vi "Project_2_VI.vi"() -> ()   [LabVIEW 2018]
doc: "I. Description:\nThis example demonstrates how to continuously acquire and generate data at the same time, synchronized with one another.\n\nII. Instructions for Running:\n1. Select the physical channel to correspond to where your signal is input on the DAQ device. Also, select the corresponding channel for where your signal is being generated.\n2. Enter the minimum and maximum voltage ranges.\nNote: For better accuracy try to match the input range to the expected voltage level of the measured signal.\n3. Set the sample rate of the acquisition.\nNote: The rate should be at least twice as fast as the maximum frequency component of the signal being acquired. \n6. Select the Rate for the generation\n7. Select what type of signal to generate and the amplitude.\nNote: This example requires two DMA channels to run. If your hardware does not support two DMA channels, you need to set the Data Transfer Mechanism property for the Analog Output Task to use \"Interrupts\". The Data Transfer Mechanism property is located in the DAQmx Channel Property hierarchy at:\n\nDAQmx Channel Property Node>>Analog Output>>General Properties>>Advanced>>Data Transfer and Memory>>Data Transfer Mechanism\n\nRefer to your device documentation to determine how many DMA channels are supported for your hardware.\n\nIII. Block Diagram Steps:\n1. Create an analog input voltage channel. Also, create an analog output voltage channel.\n2. Set the rate for the sample clock. Additionally, define the sample mode to be continuous. Also, set the sample clock rate for the signal generation.\n2a. Call the Get Terminal Name with Device Prefix VI. This will take a Task and a terminal and create a properly formatted device + terminal name to use as the source of the Trigger.\n3. Define the parameters for a Digital Edge Start Trigger. Set the Analog output to trigger off the AI Start Trigger. This is an internal trigger signal.\n4. Use the Basic Function Generator VI to create the signal to be generated.\n5. Call the Start VI to arm the two functions. Make sure the analog output is armed before the analog input. This will ensure both will start at the same time.\n6. Read the waveform data in a loop until the user hits the stop button or an error occurs. The Is Task Done? VI is used to check for errors in the Analog Output Task.\n7. Call the Clear VI to Clear the Task\n8. Use the popup dialog box to display an error if any.\n\nIV. I/O Connections Overview:\nMake sure your signal input/output terminals match the Physical Channel I/O controls."
uses:
  <vilib>/Analysis/4window.llb/windowTd.ctl
  <vilib>/Utility/error.llb/DialogType.ctl
  <vilib>/DAQmx/write.llb/DAQmx Write (Analog Wfm 1Chan NSamp).vi
  <vilib>/DAQmx/read.llb/DAQmx Read (Analog 1D Wfm NChan NSamp).vi
  <vilib>/DAQmx/create/channels.llb/DAQmx Create Channel (AI-Voltage-Basic).vi
  <vilib>/DAQmx/configure/timing.llb/DAQmx Timing (Sample Clock).vi
  <vilib>/DAQmx/create/channels.llb/DAQmx Create Channel (AO-Voltage-Basic).vi
  <vilib>/DAQmx/configure/trigger.llb/DAQmx Start Trigger (Digital Edge).vi
  <vilib>/DAQmx/miscellaneous.llb/DAQmx Fill In Error Info.vi
  <vilib>/Utility/file.llb/Write To Spreadsheet File (DBL).vi
  <vilib>/measure/maspectr.llb/FFT Spectrum (Mag-Phase) for 1 Chan.vi
  <vilib>/Utility/file.llb/Write Delimited Spreadsheet (DBL).vi
  <resource>/objmgr/daqmx.rc
  <vilib>/Analysis/NI_AALBase.lvlib
  <vilib>/measure/NI_MAPro.lvlib
  <vilib>/Analysis/NI_AALPro.lvlib
panel:
  in  "Frequency Response fike path":path=path "E:/Project2/Response.txt"
  in  "averaging parameters":T1={"averaging mode"=enum."No averaging", "weighting mode"=enum."Exponential", "number of averages"=10} {"number of averages" min=1}
  out "Phase Response":cluster{"f0":dbl, "df":dbl, "magnitude":dbl[]}(graph)
  out "Frequency Response":cluster{"f0":dbl, "df":dbl, "magnitude":dbl[]}(graph)
  in  "window":T2 items=["Rectangle"=0, "Hanning"=1, "Hamming"=2, "Blackman-Harris"=3, "Exact Blackman"=4, "Blackman"=5, "Flat Top"=6, "4 Term B-Harris "=7, "7 Term B-Harris"=8, "Low Sidelobe"=9, "Blackman Nuttall"=11, "Triangle"=30, "Bartlett-Hanning"=31, "Bohman"=32, "Parzen"=33, "Welch"=34, "Kaiser"=60, "Dolph-Chebyshev"=61, "Gaussian"=62]
  in  "End frequency (Hz)":dbl=10000.0 format="%.2p"
  in  "Waveform file path":path=path "E:/Project2/data.txt"
  in  "Start frequency":dbl=100.0 format="%0.2p"
  out "Time Domain":waveform(dbl)[](graph)
  in  "Sampling Info":T3={"Sampling Rate"=20000.0, "Number of Samples"=2000} {"Sampling Rate" format="%.2p"}
  in  "Amplitude":dbl=2.0 format="%0.2p"
  in  "Channel":tag="Dev1/ao0" caption="Output Physical Channels"
  in  "Channel":tag="Dev1/ai6,Dev1/ai13" caption="Input Physical Channel"
  # "Channel Parameters"
  # "Signal Generation"
  # "ReIm"
  # "MagPhase"
  # "FRF parameters"
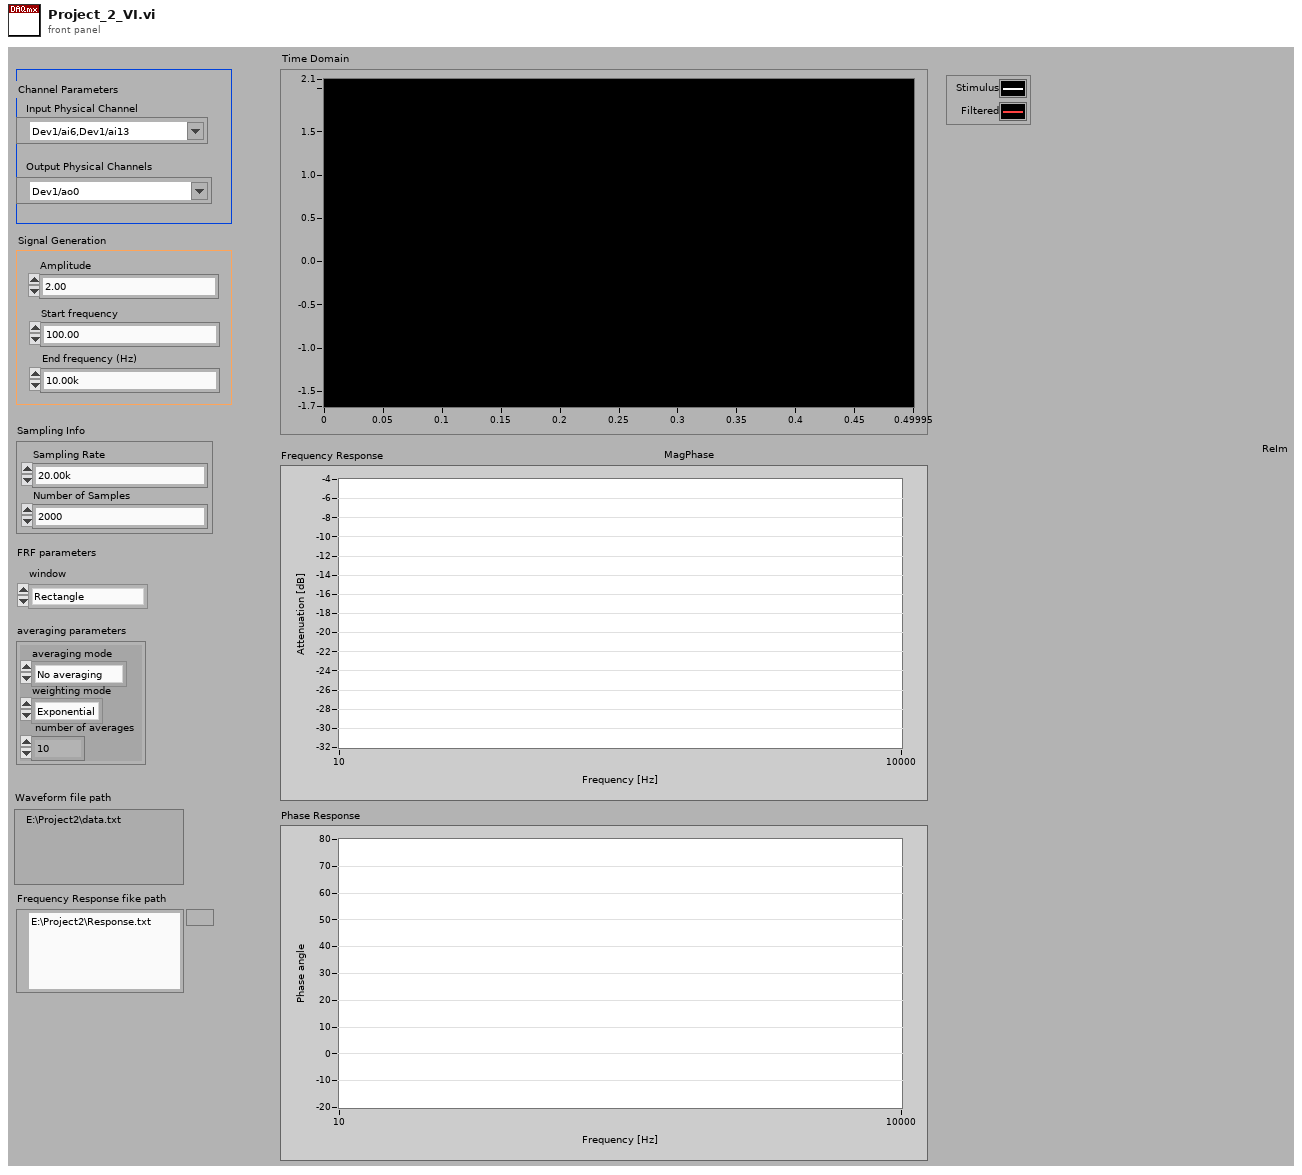
[diagram p1: front panel]
types:
  T1 = cluster{"averaging mode":enum16{"No averaging", "Vector averaging", "RMS averaging", "Peak hold"}, "weighting mode":enum16{"Linear", "Exponential"}, "number of averages":u32}
  T2 = typedef "NI_AALPro.lvlib/windowTd.ctl" = u32
  T3 = cluster{"Sampling Rate":dbl, "Number of Samples":u32}
  T4 = typedef "DialogType.ctl" = u16
  T5 = cluster{"dB On (F)":bool, "unwrap phase (F)":bool, "convert to degree (F)":bool}
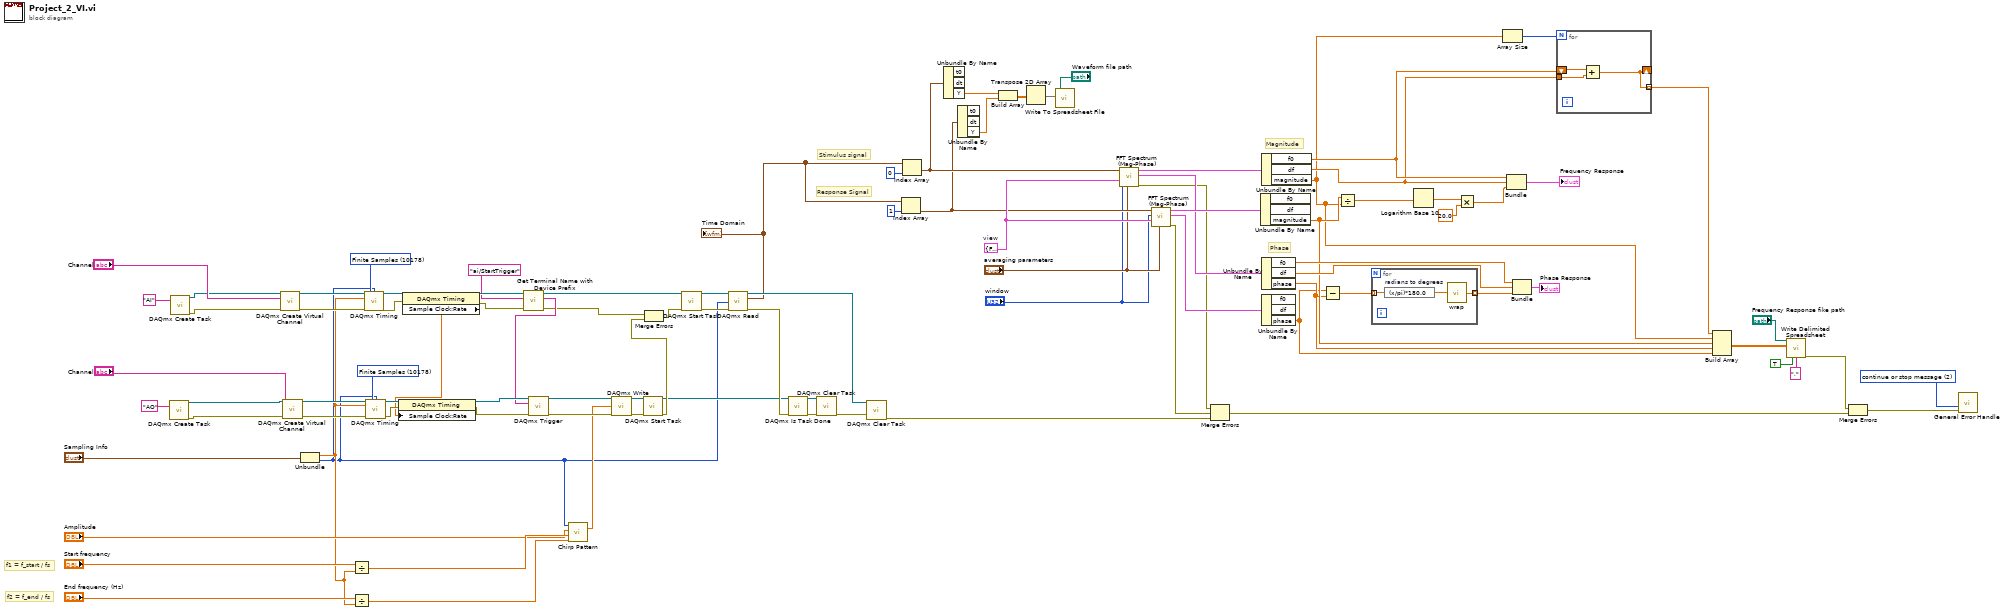
[diagram p0: block diagram]
diagram:
  w5 = T4 2 items=["no dialog", "OK message", "continue or stop message", "OK message + warnings", "continue/stop + warnings"] ("type of dialog (OK msg:1)")
  w29 = T5 {"dB On (F)"=FALSE, "unwrap phase (F)"=FALSE, "convert to degree (F)"=FALSE}  # view
  w73 = 10178 items=["Finite Samples"=10178, "Continuous Samples"=10123] ("sample mode")
  w69 = 10178 items=["Finite Samples"=10178, "Continuous Samples"=10123] ("sample mode")
  # "Phase"
  # "Magnitude"
  # "Response Signal"
  # "Stimulus signal"
  # "f2 = f_end / fs"
  # "f1 = f_start / fs"
  n1 = call <vilib>:"DAQmx Create Task.vi"("new task name"="AO") -> ("task out"=w45:refnum<k21>, "error out"=w44:errorcluster)  [unwired: 13 in]
  n2 = call <vilib>:"DAQmx Create Task.vi"("new task name"="AI") -> ("task out"=w42:refnum<k21>, "error out"=w43:errorcluster)  [unwired: 13 in]
  n3 = call-poly <vilib>:"DAQmx Create Virtual Channel.vi"("task in"=w42, "physical channels"="Channel", "error in"=w43) -> ("task out"=w71:refnum<k21>, "error out"=w70:errorcluster)  [unwired: 11 in]
  n4 = call-poly <vilib>:"DAQmx Create Virtual Channel.vi"("task in"=w45, "physical channels"="Channel", "error in"=w44) -> ("task out"=w74:refnum<k21>, "error out"=w75:errorcluster)  [unwired: 11 in]
  n5 = Unbundle("Sampling Info") -> ("Sampling Rate"=w48:dbl, "Number of Samples"=w47:u32)
  n6 = Divide(x="Start frequency", y=w48) -> (x/y=w53:dbl)
  n7 = Divide(x="End frequency (Hz)", y=w48) -> (x/y=w52:dbl)
  n8 = call-poly <vilib>:"DAQmx Timing.vi"("task/channels in"=w71, "sample mode"=w69, "samples per channel"=w47, "rate"=w48, "error in"=w70) -> ("task out"=w91:refnum<k21>, "error out"=w92:errorcluster)  [unwired: 9 in]
  n9 = call-poly <vilib>:"DAQmx Timing.vi"("task/channels in"=w74, "sample mode"=w73, "samples per channel"=w47, "rate"=w48, "error in"=w75) -> ("task out"=w84:refnum<k21>, "error out"=w85:errorcluster)  [unwired: 9 in]
  n10 = property class="DAQmx Timing"(reference=w91, error in=w92) -> (reference out=w60:refnum<k21>, error out=w58:errorcluster, "Sample Clock:Rate"=w46:dbl)
  n11 = property class="DAQmx Timing"(reference=w84, error in=w85, "Sample Clock:Rate"=w46) -> (reference out=w83:refnum<k21>, error out=w86:errorcluster)
  n12 = call "Get Terminal Name with Device Prefix.vi"("error in"=w58, "Local Terminal Name"="ai/StartTrigger" ("terminal"), "task/channels in"=w60) -> ("error out"=w55:errorcluster, "Terminal Name with Device Prefix"=w57:tag, "task out"=w56:refnum<k21>)  [unwired: 6 in]
  n13 = call-poly <vilib>:"DAQmx Trigger.vi"("task/channels in"=w83, "source"=w57, "error in"=w86) -> ("task out"=w81:refnum<k21>, "error out"=w80:errorcluster)  [unwired: 11 in]
  n14 = call <vilib>:"Chirp Pattern.vi"("f2"=w52, "f1"=w53, "amplitude"="Amplitude", "samples"=w47) -> ("Chirp Pattern"=w49:dbl[])  [unwired: 1 out]
  n15 = call-poly <vilib>:"DAQmx Write.vi"("task/channels in"=w81, "data"=w49, "error in"=w80) -> ("task out"=w78:refnum<k21>, "error out"=w79:errorcluster)  [unwired: 10 in, 1 out]
  n16 = call <vilib>:"DAQmx Start Task.vi"("task/channels in"=w78, "error in"=w79) -> ("task out"=w76:refnum<k21>, "error out"=w88:errorcluster)  [unwired: 12 in]
  n17 = Merge Errors(w55, w88) -> (w89:errorcluster)
  n18 = call <vilib>:"DAQmx Start Task.vi"("task/channels in"=w56, "error in"=w89) -> ("task out"=w87:refnum<k21>, "error out"=w90:errorcluster)  [unwired: 12 in]
  n19 = call-poly <vilib>:"DAQmx Read.vi"("task/channels in"=w87, "number of samples per channel"=w47, "error in"=w90) -> ("task out"=w68:refnum<k21>, "data"=w39:waveform(dbl)[], "error out"=w95:errorcluster)  [unwired: 10 in]
  "Time Domain" <- w39
  n20 = call <vilib>:"DAQmx Is Task Done.vi"("task/channels in"=w76, "error in"=w95) -> ("task out"=w77:refnum<k21>, "error out"=w93:errorcluster)  [unwired: 11 in, 1 out]
  n21 = call <vilib>:"DAQmx Clear Task.vi"("task in"=w77, "error in"=w93) -> ("error out"=w94:errorcluster)  [unwired: 13 in]
  n22 = call <vilib>:"DAQmx Clear Task.vi"("task in"=w68, "error in"=w94) -> ("error out"=w13:errorcluster)  [unwired: 13 in]
  n23 = Index Array(array=w39, index=1) -> (element=w25:waveform(dbl))
  n24 = Index Array(array=w39, index=0) -> (element=w26:waveform(dbl))
  n25 = Unbundle By Name(w26) -> ("Y"=w64:dbl[])  [unwired: 2 out]
  n26 = Unbundle By Name(w25) -> ("Y"=w63:dbl[])  [unwired: 2 out]
  n27 = Build Array(w64, w63) -> (w62:dbl[][])
  n28 = Transpose 2D Array(2D array=w62) -> (transposed array=w61:dbl[][])
  n29 = call-poly <vilib>:"Write To Spreadsheet File.vi"("2D data"=w61, "file path (dialog if empty)"="Waveform file path") -> ()  [unwired: 6 in, 1 out]
  n30 = call-poly <vilib>:"FFT Spectrum (Mag-Phase).vi"("averaging parameters"="averaging parameters", "view"=w29, "window"="window", "time signal"=w26) -> ("error out"=w11:errorcluster, "phase"=w22:cluster{"f0":dbl, "df":dbl, "phase":dbl[]}, "magnitude"=w34:cluster{"f0":dbl, "df":dbl, "magnitude":dbl[]})  [unwired: 3 in, 2 out]
  n31 = call-poly <vilib>:"FFT Spectrum (Mag-Phase).vi"("averaging parameters"="averaging parameters", "view"=w29, "window"="window", "time signal"=w25) -> ("error out"=w12:errorcluster, "phase"=w31:cluster{"f0":dbl, "df":dbl, "phase":dbl[]}, "magnitude"=w35:cluster{"f0":dbl, "df":dbl, "magnitude":dbl[]})  [unwired: 3 in, 2 out]
  n32 = Merge Errors(w11, w12, w13) -> (w10:errorcluster)
  n33 = Unbundle By Name(w35) -> ("magnitude"=w21:dbl[])  [unwired: 2 out]
  n34 = Unbundle By Name(w34) -> ("f0"=w20:dbl, "df"=w19:dbl, "magnitude"=w6:dbl[])
  n35 = Unbundle By Name(w22) -> ("f0"=w27:dbl, "df"=w28:dbl, "phase"=w3:dbl[])
  n36 = Unbundle By Name(w31) -> ("phase"=w2:dbl[])  [unwired: 2 out]
  n37 = Subtract(x=w2, y=w3) -> (x-y=w30:dbl[])
  n38 = Divide(x=w21, y=w6) -> (x/y=w33:dbl[])
  n39 = for {
    tunnel: w30 -> [w98] mode=indexing
    tunnel: [w99] -> w1 mode=indexing
    n40 = expression code="(x/pi)*180.0" "radians to degrees"(w98) -> (w97:dbl)
    n41 = call "wrap.vi"("Degrees In"=w97) -> ("Degrees Out"=w99:dbl)
  }
  n42 = Logarithm Base 10(1:w33) -> (0:w38:dbl[])
  n43 = Multiply(x=w38, y=20.0) -> (x*y=w4:dbl[])
  n44 = Array Size(array=w6) -> (size(s)=w7:i32)
  n45 = Bundle("f0"=w20, "df"=w19, w4) -> (→"Frequency Response":cluster{"f0":dbl, "df":dbl, dbl[]})  [unwired: 1 in]
  n46 = Bundle("f0"=w27, "df"=w28, w1) -> (→"Phase Response":cluster{"f0":dbl, "df":dbl, dbl[]})  [unwired: 1 in]
  n47 = for {
    N: w7 -> [_]
    shift-right: [w100] -> _
    shift-left: w20 -> [w102]
    tunnel: w19 -> [w101]
    tunnel: [w100] -> w18 mode=indexing
    n48 = Add(x=w102, y=w101) -> (x+y=w100:dbl)
  }
  n49 = Build Array(w18, w6, w21, w3, w2) -> (w17:dbl[][])
  n50 = call-poly <vilib>:"Write Delimited Spreadsheet.vi"("file path (dialog if empty)"="Frequency Response fike path", "2D data"=w17, "transpose? (no:F)"=TRUE, "delimiter (\\t)"="," ("delimiter (\\t)")) -> ("error out"=w9:errorcluster)  [unwired: 10 in, 1 out]
  n51 = Merge Errors(w9, w10) -> (w8:errorcluster)
  n52 = call <vilib>:"General Error Handler.vi"("type of dialog (OK msg:1)"=w5, "error in (no error)"=w8) -> ()  [unwired: 9 in, 5 out]
